vi "WC_Drive_CheesyDriveHelper.vi"(7 "MQuickStopAccumulator":dbl format="%#_13g", 8 "KTurnSensitivity":dbl=1.6 format="%#_13g", 10 "Steer":dbl format="%#_13g", 11 "Throttle":dbl format="%#_13g") -> (2 "RightPwm Out":dbl, 3 "LeftPwm Out":dbl, 5 "MQuickStopAccumulator Out":dbl)   [LabVIEW 2017]
panel:
  in  "quick turn cutoff":dbl=0.05 format="%#_13g"
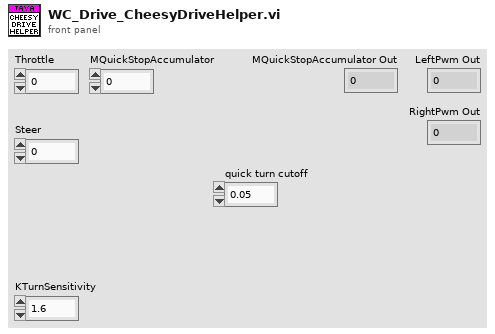
[diagram p1: front panel]
types:
  T1 = cluster{"mQuickStopAccumulator":dbl, "kThrottleDeadband":dbl, "kWheelDeadband":dbl, "kTurnSensitivity":dbl, "Steer":dbl, "Throttle":dbl, "overPower":dbl, "angularPower":dbl, "isQuickTurn":bool, "Alpha":dbl, "rightPwm":dbl, "leftPwm":dbl, "quick turn cutoff":dbl}
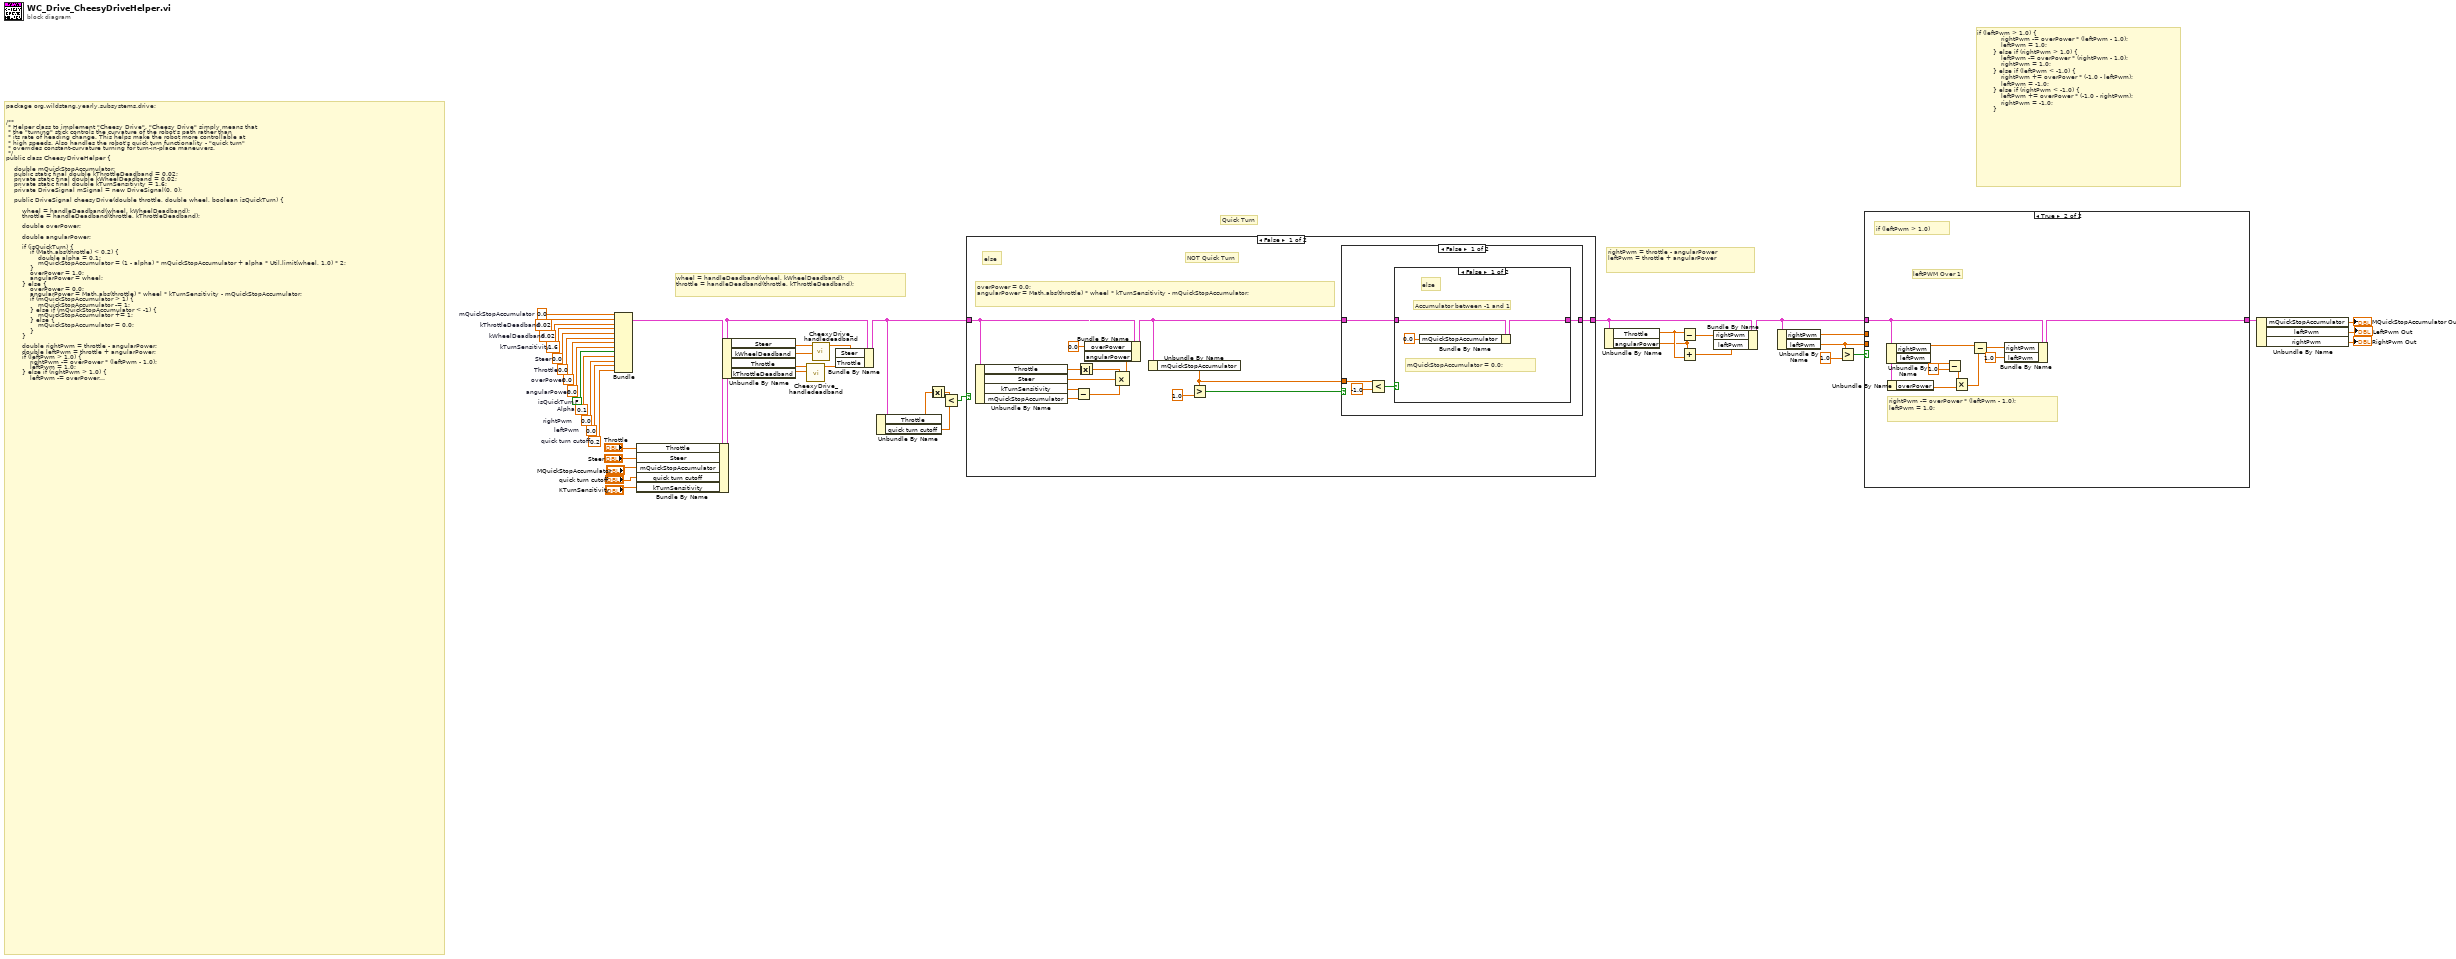
[diagram p0: block diagram]
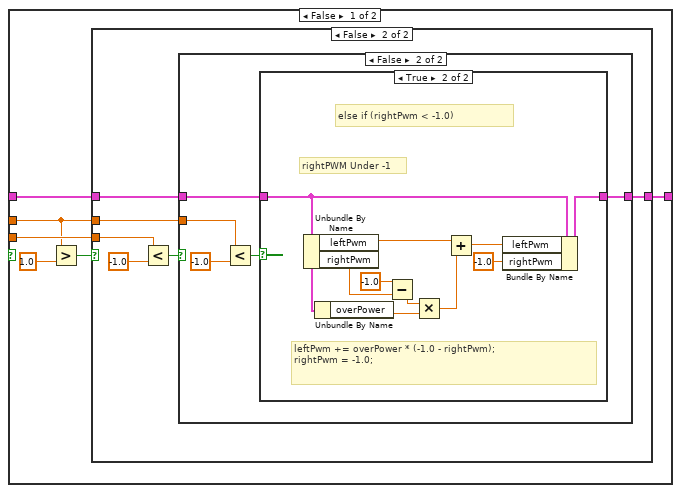
[diagram p2: hidden frame]
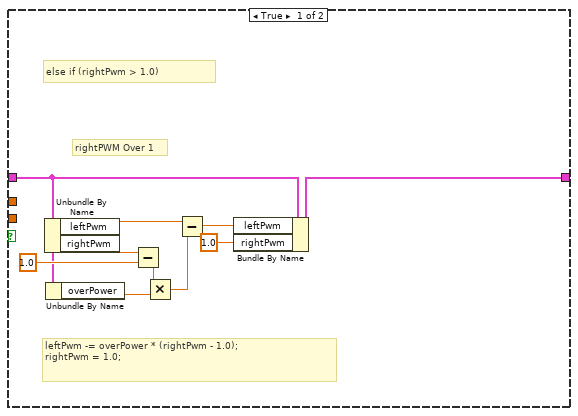
[diagram p3: hidden frame]
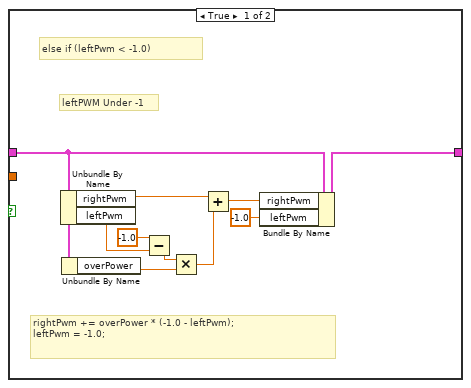
[diagram p4: hidden frame]
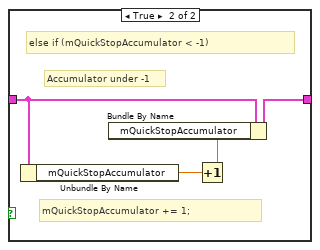
[diagram p6: hidden frame]
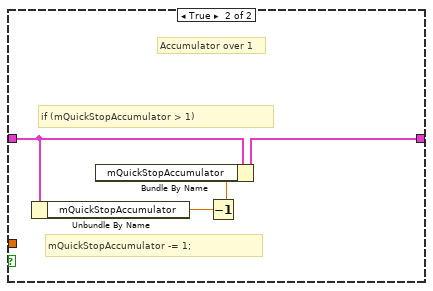
[diagram p7: hidden frame]
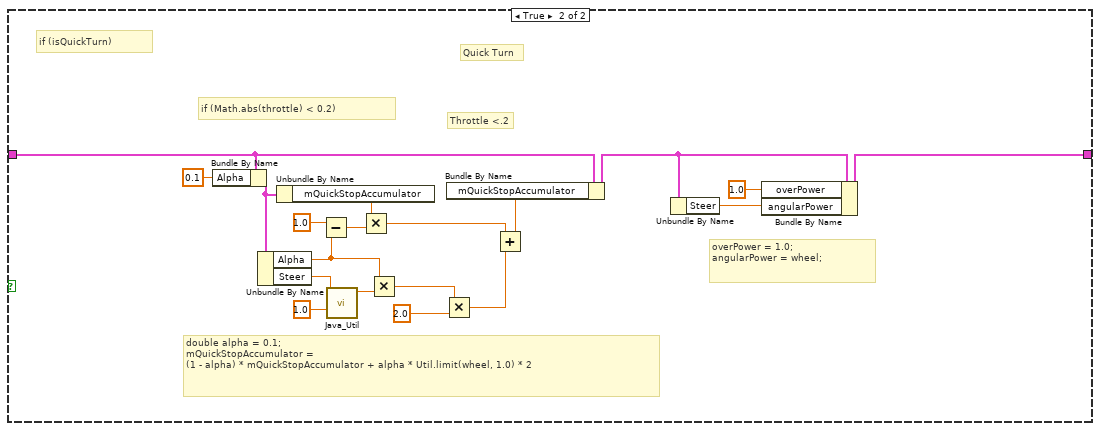
[diagram p8: hidden frame]
diagram:
  w4 = 0.2  # quick turn cutoff
  w22 = 0.0  # leftPwm
  w23 = 0.0  # rightPwm
  w36 = 0.1  # Alpha
  w37 = FALSE  # isQuickTurn
  w38 = 0.0  # angularPower
  w41 = 0.0  # Steer
  w40 = 0.0  # Throttle
  w42 = 1.6  # kTurnSensitivity
  w45 = 0.0  # mQuickStopAccumulator
  w39 = 0.0  # overPower
  w43 = 0.02  # kWheelDeadband
  w44 = 0.02  # kThrottleDeadband
  # "Quick Turn"
  # "if (leftPwm > 1.0) {\n            rightPwm -= overPower * (leftPwm - 1.0);\n            leftPwm = 1.0;\n        } else if (rightPwm > 1.0) {\n            leftPwm -= overPower * (rightPwm - 1.0);\n            rightPwm = 1.0;\n        } else if (leftPwm < -1.0) {\n            rightPwm += overPower * (-1.0 - leftPwm);\n            leftPwm = -1.0;\n        } else if (rightPwm < -1.0) {\n            leftPwm += overPower * (-1.0 - rightPwm);\n            rightPwm = -1.0;\n        }"
  # "rightPwm = throttle - angularPower\nleftPwm = throttle + angularPower"
  # "wheel = handleDeadband(wheel, kWheelDeadband);\nthrottle = handleDeadband(throttle, kThrottleDeadband);"
  # "package org.wildstang.yearly.subsystems.drive;\n\n\n/**\n * Helper class to implement \"Cheesy Drive\". \"Cheesy Drive\" simply means that\n * the \"turning\" stick controls the curvature of the robot's path rather than\n * its rate of heading change. This helps make the robot more controllable at\n * high speeds. Also handles the robot's quick turn functionality - \"quick turn\"\n * overrides constant-curvature turning for turn-in-place maneuvers.\n */\npublic class CheesyDriveHelper {\n\n    double mQuickStopAccumulator;\n    public static final double kThrottleDeadband = 0.02;\n    private static final double kWheelDeadband = 0.02;\n    private static final double kTurnSensitivity = 1.6;\n    private DriveSignal mSignal = new DriveSignal(0, 0);\n\n    public DriveSignal cheesyDrive(double throttle, double wheel, boolean isQuickTurn) {\n\n        wheel = handleDeadband(wheel, kWheelDeadband);\n        throttle = handleDeadband(throttle, kThrottleDeadband);\n\n        double overPower;\n\n        double angularPower;\n\n        if (isQuickTurn) {\n            if (Math.abs(throttle) < 0.2) {\n                double alpha = 0.1;\n                mQuickStopAccumulator = (1 - alpha) * mQuickStopAccumulator + alpha * Util.limit(wheel, 1.0) * 2;\n            }\n            overPower = 1.0;\n            angularPower = wheel;\n        } else {\n            overPower = 0.0;\n            angularPower = Math.abs(throttle) * wheel * kTurnSensitivity - mQuickStopAccumulator;\n            if (mQuickStopAccumulator > 1) {\n                mQuickStopAccumulator -= 1;\n            } else if (mQuickStopAccumulator < -1) {\n                mQuickStopAccumulator += 1;\n            } else {\n                mQuickStopAccumulator = 0.0;\n            }\n        }\n\n        double rightPwm = throttle - angularPower;\n        double leftPwm = throttle + angularPower;\n        if (leftPwm > 1.0) {\n            rightPwm -= overPower * (leftPwm - 1.0);\n            leftPwm = 1.0;\n        } else if (rightPwm > 1.0) {\n            leftPwm -= overPower * (rightPwm - 1.0);\n            rightPwm = 1.0;\n        } else if (leftPwm < -1.0) {\n            rightPwm += overPower * (-1.0 - leftPwm);\n            leftPwm = -1.0;\n        } else if (rightPwm < -1.0) {\n            leftPwm += overPower * (-1.0 - rightPwm);\n            rightPwm = -1.0;\n        }\n        mSignal.rightMotor = rightPwm;\n        mSignal.leftMotor = leftPwm;\n        return mSignal;\n    }\n\n    public double handleDeadband(double val, double deadband) {\n        return (Math.abs(val) > Math.abs(deadband)) ? val : 0.0;\n    }\n}"
  n1 = Bundle("mQuickStopAccumulator"=w45, "kThrottleDeadband"=w44, "kWheelDeadband"=w43, "kTurnSensitivity"=w42, "Steer"=w41, "Throttle"=w40, "overPower"=w39, "angularPower"=w38, "isQuickTurn"=w37, "Alpha"=w36, "rightPwm"=w23, "leftPwm"=w22, "quick turn cutoff"=w4) -> (w27:T1)  [unwired: 1 in]
  n2 = Bundle By Name(cluster=w27, "Throttle"="Throttle", "Steer"="Steer", "mQuickStopAccumulator"="MQuickStopAccumulator", "quick turn cutoff"="quick turn cutoff", "kTurnSensitivity"="KTurnSensitivity") -> (w26:T1)
  n3 = Unbundle By Name(w26) -> ("Steer"=w33:dbl, "kWheelDeadband"=w32:dbl, "Throttle"=w31:dbl, "kThrottleDeadband"=w30:dbl)
  n4 = call "CheexyDrive_handledeadband.vi"("Deadband"=w30, "val"=w31) -> ("Val Out"=w28:dbl)  [unwired: 9 in]
  n5 = call "CheexyDrive_handledeadband.vi"("Deadband"=w32, "val"=w33) -> ("Val Out"=w29:dbl)  [unwired: 9 in]
  n6 = Bundle By Name(cluster=w26, "Steer"=w29, "Throttle"=w28) -> (w5:T1)
  n7 = Unbundle By Name(w5) -> ("Throttle"=w7:dbl, "quick turn cutoff"=w2:dbl)
  n8 = Absolute Value(x=w7) -> (abs(x)=w8:dbl)
  n9 = Less?(x=w8, y=w2) -> (x < y?=w6:bool)
  n10 = case shown="False" w6 {
    tunnel: w5 -> [w51 w94]
    tunnel: [w50 w93] -> w21
    frame False {
      # "NOT Quick Turn"
      # "overPower = 0.0;\nangularPower = Math.abs(throttle) * wheel * kTurnSensitivity - mQuickStopAccumulator;"
      # "else"
      n11 = Unbundle By Name(w51) -> ("Throttle"=w57:dbl, "Steer"=w55:dbl, "kTurnSensitivity"=w58:dbl, "mQuickStopAccumulator"=w59:dbl)
      n12 = Subtract(x=w58, y=w59) -> (x-y=w54:dbl)
      n13 = Absolute Value(x=w57) -> (abs(x)=w56:dbl)
      n14 = Compound Arithmetic op=MULTIPLY(w56, w55, w54) -> (w53:dbl)
      n15 = Bundle By Name(cluster=w51, "overPower"=0.0, "angularPower"=w53) -> (w49:T1)
      n16 = Unbundle By Name(w49) -> ("mQuickStopAccumulator"=w46:dbl)
      n17 = Greater?(x=w46, y=1.0) -> (0:w47:bool)
      n18 = case shown="False" w47 {
        tunnel: w49 -> [w61 w75]
        tunnel: [w60 w74] -> w50
        tunnel: w46 -> [w64 _]
        frame False {
          n19 = Less?(x=w64, y=-1.0) -> (x < y?=w62:bool)
          n20 = case shown="False" w62 {
            tunnel: w61 -> [w67 w69]
            tunnel: [w66 w68] -> w60
            frame False {
              # "else"
              # "Accumulator between -1 and 1"
              # "mQuickStopAccumulator = 0.0;"
              n21 = Bundle By Name(cluster=w67, "mQuickStopAccumulator"=0.0) -> (w66:T1)
            }
            frame True {
              # "Accumulator under -1"
              # "mQuickStopAccumulator += 1;"
              # "else if (mQuickStopAccumulator < -1)"
              n22 = Unbundle By Name(w69) -> ("mQuickStopAccumulator"=w71:dbl)
              n23 = Increment(x=w71) -> (x+1=w70:dbl)
              n24 = Bundle By Name(cluster=w69, "mQuickStopAccumulator"=w70) -> (w68:T1)
            }
          }
        }
        frame True {
          # "Accumulator over 1"
          # "if (mQuickStopAccumulator > 1)"
          # "mQuickStopAccumulator -= 1;"
          n25 = Unbundle By Name(w75) -> ("mQuickStopAccumulator"=w73:dbl)
          n26 = Decrement(x=w73) -> (x-1=w72:dbl)
          n27 = Bundle By Name(cluster=w75, "mQuickStopAccumulator"=w72) -> (w74:T1)
        }
      }
    }
    frame True {
      # "Throttle <.2"
      # "double alpha = 0.1;\nmQuickStopAccumulator = \n(1 - alpha) * mQuickStopAccumulator + alpha * Util.limit(wheel, 1.0) * 2"
      # "if (Math.abs(throttle) < 0.2)"
      # "Quick Turn"
      # "overPower = 1.0;\nangularPower = wheel;"
      # "if (isQuickTurn)"
      n28 = Bundle By Name(cluster=w94, "Alpha"=0.1) -> (w82:T1)
      n29 = Unbundle By Name(w82) -> ("Alpha"=w83:dbl, "Steer"=w80:dbl)
      n30 = Unbundle By Name(w82) -> ("mQuickStopAccumulator"=w81:dbl)
      n31 = Subtract(x=1.0, y=w83) -> (x-y=w88:dbl)
      n32 = call "Java_Util.vi"("Limit"=1.0, "V"=w80) -> ("V Out"=w86:dbl)  [unwired: 9 in]
      n33 = Multiply(x=w81, y=w88) -> (x*y=w85:dbl)
      n34 = Multiply(x=w83, y=w86) -> (x*y=w78:dbl)
      n35 = Multiply(x=w78, y=2.0) -> (x*y=w77:dbl)
      n36 = Add(x=w85, y=w77) -> (x+y=w76:dbl)
      n37 = Bundle By Name(cluster=w94, "mQuickStopAccumulator"=w76) -> (w91:T1)
      n38 = Unbundle By Name(w91) -> ("Steer"=w90:dbl)
      n39 = Bundle By Name(cluster=w91, "overPower"=1.0, "angularPower"=w90) -> (w93:T1)
    }
  }
  n40 = Unbundle By Name(w21) -> ("Throttle"=w20:dbl, "angularPower"=w19:dbl)
  n41 = Subtract(x=w20, y=w19) -> (x-y=w18:dbl)
  n42 = Add(x=w19, y=w20) -> (x+y=w17:dbl)
  n43 = Bundle By Name(cluster=w21, "rightPwm"=w18, "leftPwm"=w17) -> (w15:T1)
  n44 = Unbundle By Name(w15) -> ("rightPwm"=w12:dbl, "leftPwm"=w11:dbl)
  n45 = Greater?(x=w11, y=1.0) -> (0:w13:bool)
  n46 = case shown="True" w13 {
    tunnel: w15 -> [w98 w147]
    tunnel: [w97 w152] -> w16
    tunnel: w12 -> [w95 _]
    tunnel: w11 -> [w96 _]
    frame False {
      n47 = Greater?(x=w95, y=1.0) -> (0:w99:bool)
      n48 = case shown="False" w99 {
        tunnel: w98 -> [w102 w116]
        tunnel: [w101 w115] -> w97
        tunnel: w96 -> [_ w113]
        tunnel: w95 -> [_ w111]
        frame True {
          # "rightPWM Over 1"
          # "leftPwm -= overPower * (rightPwm - 1.0);\nrightPwm = 1.0;"
          # "else if (rightPwm > 1.0)"
          n49 = Unbundle By Name(w102) -> ("leftPwm"=w110:dbl, "rightPwm"=w107:dbl)
          n50 = Unbundle By Name(w102) -> ("overPower"=w104:dbl)
          n51 = Subtract(x=w107, y=1.0) -> (x-y=w105:dbl)
          n52 = Multiply(x=w105, y=w104) -> (x*y=w103:dbl)
          n53 = Subtract(x=w110, y=w103) -> (x-y=w109:dbl)
          n54 = Bundle By Name(cluster=w102, "leftPwm"=w109, "rightPwm"=1.0 ("leftPwm")) -> (w101:T1)
        }
        frame False {
          n55 = Less?(x=w113, y=-1.0) -> (x < y?=w112:bool)
          n56 = case shown="False" w112 {
            tunnel: w116 -> [w118 w131]
            tunnel: [w117 w130] -> w115
            tunnel: w111 -> [_ w128]
            frame True {
              # "leftPWM Under -1"
              # "rightPwm += overPower * (-1.0 - leftPwm);\nleftPwm = -1.0;"
              # "else if (leftPwm < -1.0)"
              n57 = Unbundle By Name(w118) -> ("rightPwm"=w126:dbl, "leftPwm"=w123:dbl)
              n58 = Unbundle By Name(w118) -> ("overPower"=w120:dbl)
              n59 = Subtract(x=-1.0 ("y"), y=w123) -> (x-y=w121:dbl)
              n60 = Multiply(x=w121, y=w120) -> (x*y=w119:dbl)
              n61 = Add(x=w126, y=w119) -> (x+y=w125:dbl)
              n62 = Bundle By Name(cluster=w118, "rightPwm"=w125, "leftPwm"=-1.0) -> (w117:T1)
            }
            frame False {
              n63 = Less?(x=w128, y=-1.0) -> (x < y?=w127:bool)
              n64 = case shown="True" w127 {
                tunnel: w131 -> [w132 w134]
                tunnel: [w132 w133] -> w130
                frame False {
                  # "Both PWMs between -1 and 1"
                }
                frame True {
                  # "rightPWM Under -1"
                  # "leftPwm += overPower * (-1.0 - rightPwm);\nrightPwm = -1.0;"
                  # "else if (rightPwm < -1.0)"
                  n65 = Unbundle By Name(w134) -> ("leftPwm"=w142:dbl, "rightPwm"=w139:dbl)
                  n66 = Unbundle By Name(w134) -> ("overPower"=w136:dbl)
                  n67 = Subtract(x=-1.0 ("y"), y=w139) -> (x-y=w137:dbl)
                  n68 = Multiply(x=w137, y=w136) -> (x*y=w135:dbl)
                  n69 = Add(x=w142, y=w135) -> (x+y=w141:dbl)
                  n70 = Bundle By Name(cluster=w134, "leftPwm"=w141, "rightPwm"=-1.0 ("leftPwm")) -> (w133:T1)
                }
              }
            }
          }
        }
      }
    }
    frame True {
      # "leftPWM Over 1"
      # "rightPwm -= overPower * (leftPwm - 1.0);\nleftPwm = 1.0;"
      # "if (leftPwm > 1.0)"
      n71 = Unbundle By Name(w147) -> ("rightPwm"=w151:dbl, "leftPwm"=w148:dbl)
      n72 = Unbundle By Name(w147) -> ("overPower"=w144:dbl)
      n73 = Subtract(x=w148, y=1.0) -> (x-y=w145:dbl)
      n74 = Multiply(x=w145, y=w144) -> (x*y=w143:dbl)
      n75 = Subtract(x=w151, y=w143) -> (x-y=w150:dbl)
      n76 = Bundle By Name(cluster=w147, "rightPwm"=w150, "leftPwm"=1.0) -> (w152:T1)
    }
  }
  n77 = Unbundle By Name(w16) -> ("mQuickStopAccumulator"=→"MQuickStopAccumulator Out":dbl, "leftPwm"=→"LeftPwm Out":dbl, "rightPwm"=→"RightPwm Out":dbl)
